vi "my own integrator.vi"(7 "initialize":bool, 9 "dt":dbl=1.0 format="%0.2f", 10 "initial condition":dbl format="%0.2f", 11 "x":dbl format="%0.2f") -> (3 "integral x(t)":dbl format="%0.2f")   [LabVIEW 2014, in "UEGO Sim Engine.lvlib"]
uses:
  UEGO Sim Engine.lvlib
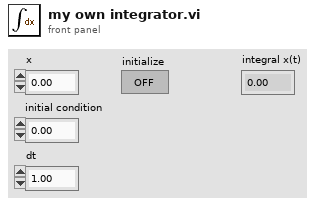
[diagram p1: front panel]
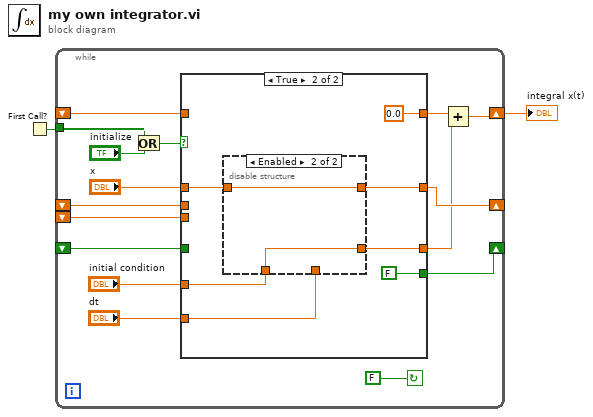
[diagram p0: block diagram]
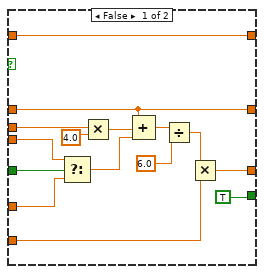
[diagram p2: hidden frame]
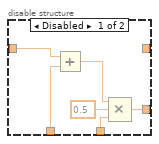
[diagram p3: hidden frame]
diagram:
  n1 = First Call?() -> (First Call?: T/F=w2:bool)
  n2 = while {
    shift-left: _ -> [w6]
    shift-right: [w3] -> w1
    tunnel: w2 -> [w15]
    shift-left: _ -> [w10]
    shift-right: [w18] -> _
    shift-left: _ -> [w8]
    shift-left: _ -> [w9]
    shift-right: [w12] -> _
    stop <- FALSE continue-if-true
    n3 = Or(x=w15, y="initialize") -> (x .or. y?=w14:bool)
    n4 = case shown="True" w14 {
      tunnel: [TRUE FALSE ("Boolean")] -> w18
      tunnel: "dt" -> [w32 w36]
      tunnel: "x" -> [w29 w37]
      tunnel: [w29 w34] -> w12
      tunnel: "initial condition" -> [w20 w35]
      tunnel: [w31 w40] -> w4
      tunnel: w10 -> [w22 _]
      tunnel: w9 -> [w33 _]
      tunnel: w8 -> [w21 _]
      tunnel: [w28 0.0] -> w5
      tunnel: w6 -> [w28 _]
      frame False {
        n5 = Select(t=w21, s=w22, f=w20) -> (s? t:f=w19:dbl)
        n6 = Multiply(x=w33, y=4.0) -> (x*y=w26:dbl)
        n7 = Compound Arithmetic op=ADD(w29, w26, w19) -> (w25:dbl)
        n8 = Divide(x=w25, y=6.0) -> (x/y=w23:dbl)
        n9 = Multiply(x=w23, y=w32) -> (x*y=w31:dbl)
      }
      frame True {
        n10 = disable-structure shown="Enabled" {
          disable-tunnel: [w46 w48] -> w40
          disable-tunnel: w37 -> [w45 w47]
          disable-tunnel: w36 -> [w42 _]
          disable-tunnel: w35 -> [w41 w48]
          disable-tunnel: [_ w47] -> w34
          frame Disabled {
            n11 = Add(x=w45, y=w41) -> (x+y=w44:dbl)
            n12 = Compound Arithmetic op=MULTIPLY(w44, 0.5 ("Input"), w42) -> (w46:dbl)
          }
          frame Enabled {
          }
        }
      }
    }
    n13 = Add(x=w5, y=w4) -> (x+y=w3:dbl)
  }
  "integral x(t)" <- w1
